vi "GlueSingleModule(SubVI).vi"(0 "XYZ Stage Control":refnum<k24>, 1 "Template Path":path=path "C:/Users/Aerotech/Documents/BNL_ThermomechanicalStave/1_ModulePlacement", 3 "Image Feed":T7, 5 "Module corner coordinates":T3={"X [mm]"=300.0, "Y [mm]"=-149.0, "Z [mm] "=-49.0}, 9 "um/pix resolution":dbl=1.5800403213058958, 11 "error in":errorcluster, 12 "Calibrate distance?":bool, 13 "Tape Type":T2=enum."Left stereo", 14 "Path to save collected images":path=path "C:/Users/Aerotech/cernbox/BNL/Stave Assembly Records/2017-05-12") -> (4 "XYZ .NET Refnum out":refnum<k24>, 15 "error out":errorcluster={"status"=FALSE, "code"=1073676418, "source"="VISA Close in GlueSingleModule(SubVI).vi"})   [LabVIEW 2016]
uses:
  C:/Users/Aerotech/Documents/BNL_ThermomechanicalStave/AerotechLibraries/Bin/Aerotech.A3200.dll
  AerotechLibraries/Bin/Aerotech.A3200.dll
  <vilib>/LabVIEW Interface for Arduino/Type Defs/Arduino Resource.ctl
  <vilib>/LabVIEW Interface for Arduino/Type Defs/Board Type.ctl
  Utils/Enum_TypeDefinitions/Enum_TypeDef_TapeType.ctl
  <vilib>/vision/Image Controls.llb/IMAQ Image.ctl
  <vilib>/LabVIEW Interface for Arduino/Type Defs/Pin Mode.ctl
  <vilib>/Utility/file.llb/Read Delimited Spreadsheet (DBL).vi
  <vilib>/LabVIEW Interface for Arduino/LabVIEW Interface for Arduino.lvlib
panel:
  in  "?":T1(tab)
  in  "Axis speeds (mm/s)":T4={"vX [mm]"=49.0, "vY [mm]"=49.0, "vZ [mm] "=49.0}
  in  "Module length [mm] Y":dbl=90.0
  in  "Module width [mm] X":dbl=90.0
  in  "Home?":bool
  in  "Lowest Z Position":dbl=-47.0
  out "Arduino Resource":T5={"VISA resource"="COM4", "Board Type"=enum."Uno", "Connection Type"=enum."USB / Serial", "Bytes Per Packet (15)"=15}
  in  "Digital I/O Pin":u8=7
  in  "Testing?":bool
  out "Difference camera/syringe in X":dbl
  out "Difference camera/syringe in y":dbl
  in  "Highest Z position":dbl=-49.0
  out "INPUT : Dot":bool[][](array[boolean])
  out "Row":i32
  out "Column":i32
  out "Final Position":T8={"Final X"=300.0000050817871, "Final Y"=-148.9999969595597, "Final Z"=-48.99995500508501}
  out "DY [mm]":dbl[](array[numeric])
  out "DX [mm]":dbl[](array[numeric])
  # "DISPENSE GLUE FOR ONE MODULE  Brandeis University - Brookhaven National Laboratory * ATLAS Phase II Inner Tracker Upgrade"
  # "Overview: This takes a pattern of zeroes/ones (.csv file) as well as the start coordinates of the top left corner of a module and places dots of glue  \nRequirements: NI Arduino dependencies\nInstructions: Select a .csv file (ones indicate regions for glue) as well as a starting coordinate (this is default to the top left corner of the module spacer). You \ncan also input axis speeds (default to maximum) and module lengths and widths (default to 90 mm) which are the widths of the module to which you want to \nplace glue. Lastly, one can choose to Home the stage here and can select the lowest position in Z. The default is that the stage moves down 2-3 mm in Z \nwhile dispensing.  The Arduino inputs are default and simply allow the LabView program to drigger the Arduino (which sends a signal to the dispenser). The \nprogram signals to dispense air- all other parameters such as length of dispensing (default: 350 millisec), pressure (default: 48 psi), and vacuum pressure \n(default: 7.8 psi) are set on the dispenser itself. The defaults are highly recommended here."
  # "Positioning Inputs"
  # "Arduino Inputs"
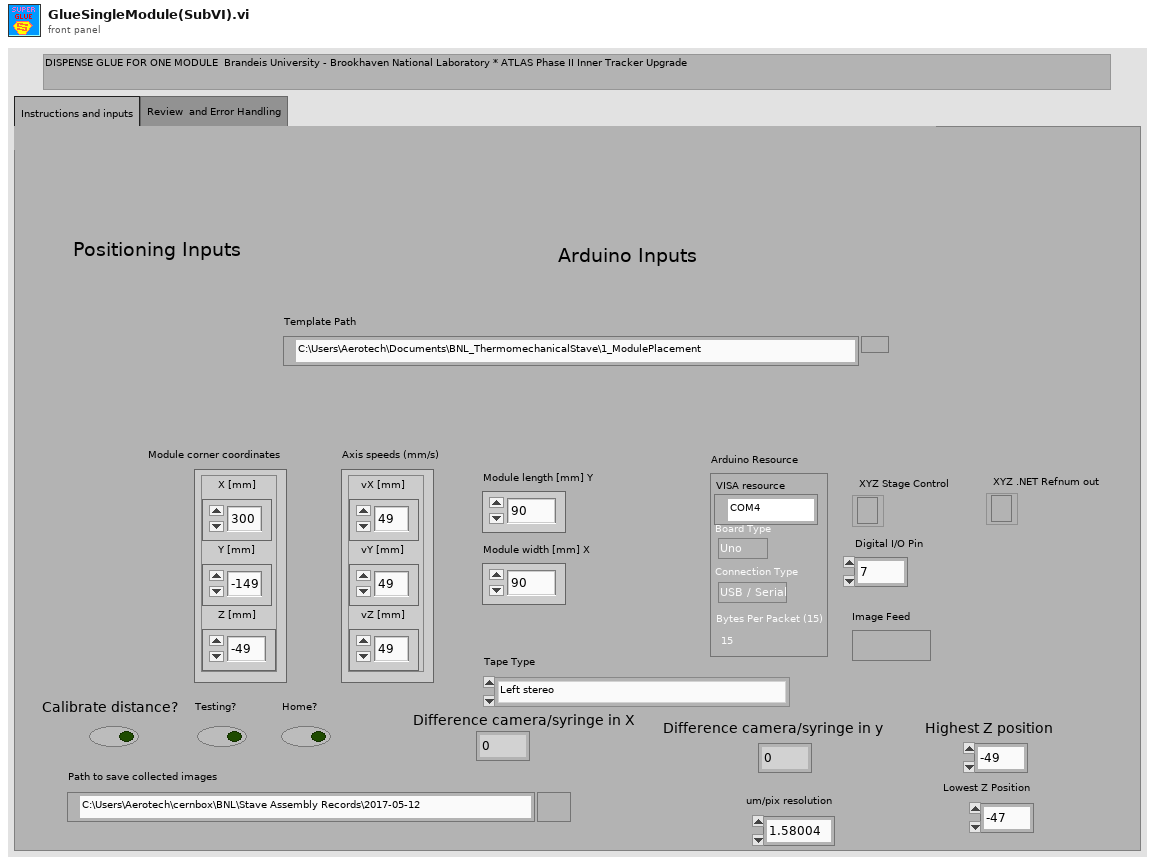
[diagram p1: front panel]
types:
  T1 = enum32{"Instructions and inputs", "Review  and Error Handling"}
  T2 = typedef "Enum_TypeDef_TapeType.ctl" = enum16{"Right stereo", "Left stereo", "Stereo (Sutcliffe NP49-01-100 01-Mar-16)", "Axial (Sutcliffe NP49-01-100 01-Mar-16)"}
  T3 = cluster{"X [mm]":dbl, "Y [mm]":dbl, "Z [mm] ":dbl}
  T4 = cluster{"vX [mm]":dbl, "vY [mm]":dbl, "vZ [mm] ":dbl}
  T5 = typedef "LabVIEW Interface for Arduino.lvlib/Arduino Resource.ctl" = cluster{"VISA resource":refnum<visa-resource-name>, "Board Type":T6, "Connection Type":enum8{"USB / Serial"}, "Bytes Per Packet (15)":u8}
  T6 = typedef "LabVIEW Interface for Arduino.lvlib/Board Type.ctl" = enum16{"Uno", "Dimuelanove w/Atmega 328", "Mega 2560"}
  T7 = typedef "IMAQ Image.ctl" = refnum<image>
  T8 = cluster{"Final X":dbl, "Final Y":dbl, "Final Z":dbl}
  T9 = typedef "LabVIEW Interface for Arduino.lvlib/Pin Mode.ctl" = enum8{"Input", "Output"}
  T10 = cluster{"Final Y":dbl, "Final Y":dbl, "Final Z":dbl}
  T11 = cluster{"Final X":dbl, "Final Y":dbl, "Lowest Z Position":dbl}
  T12 = cluster{"Final X":dbl, "Final Y":dbl, "Z [mm] ":dbl}
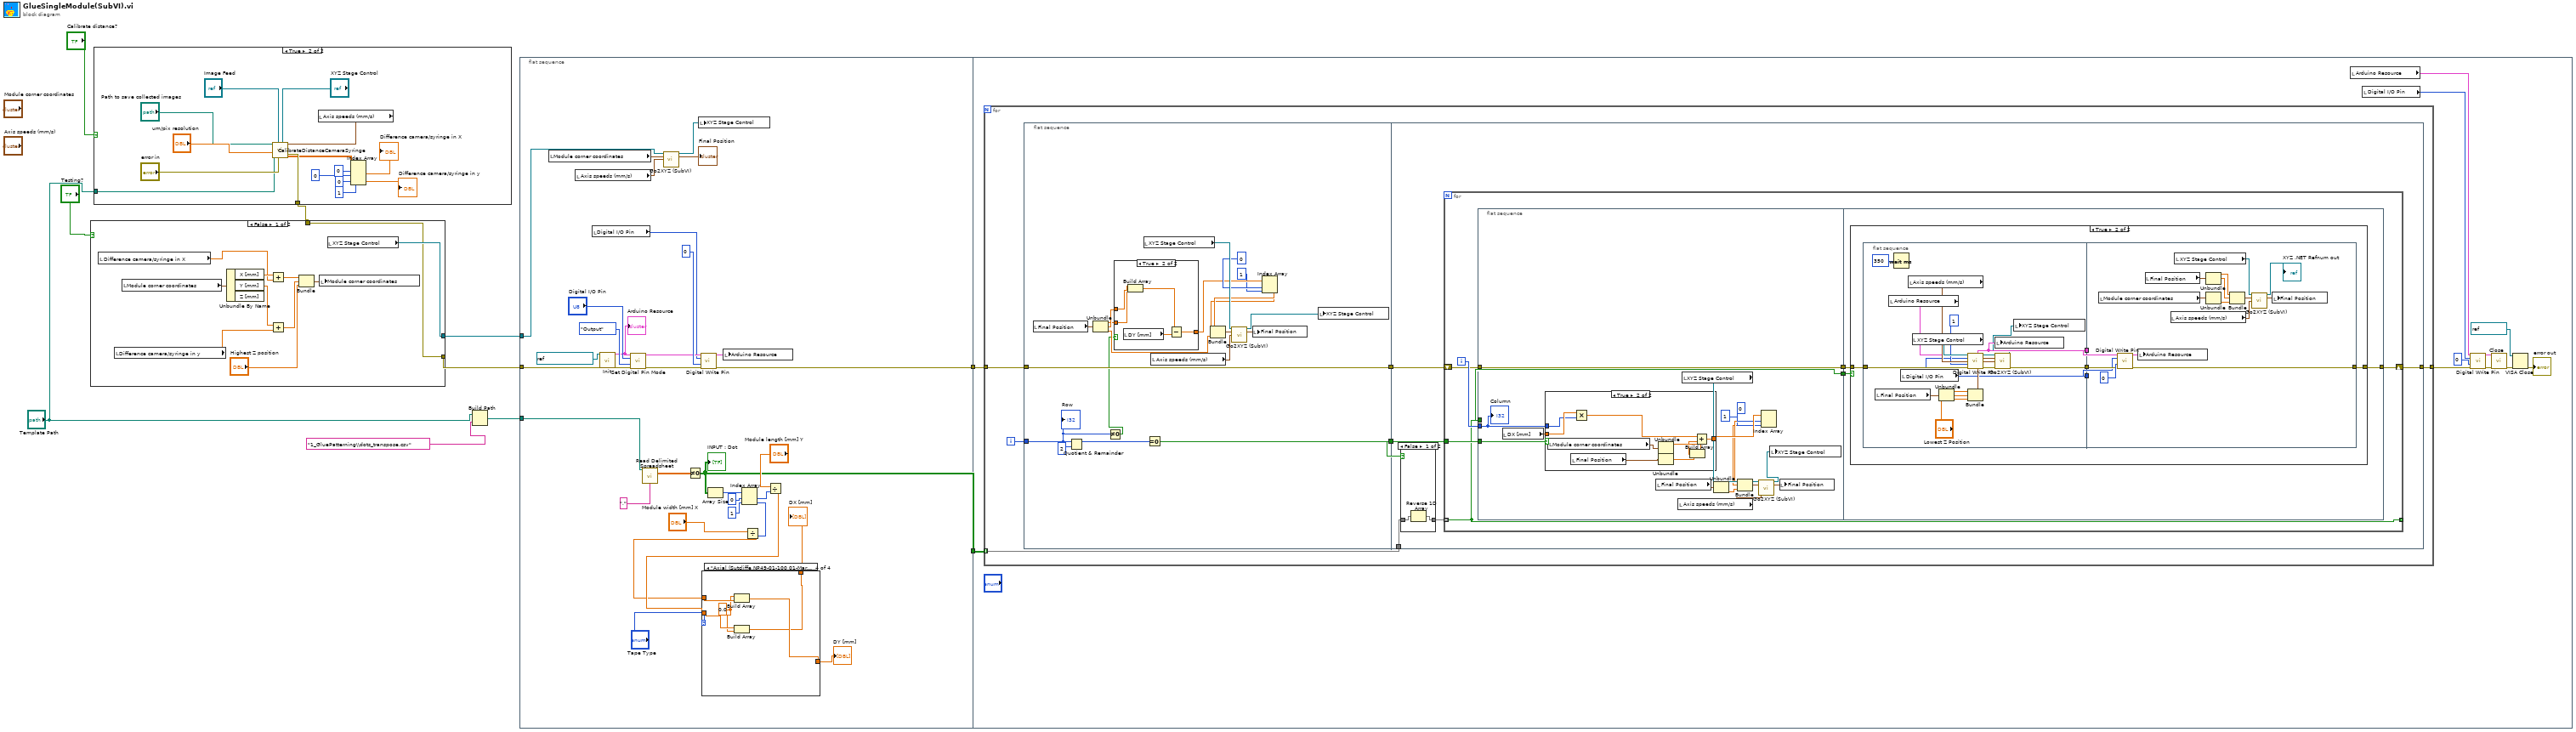
[diagram p0: block diagram]
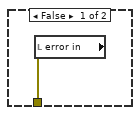
[diagram p2: hidden frame]
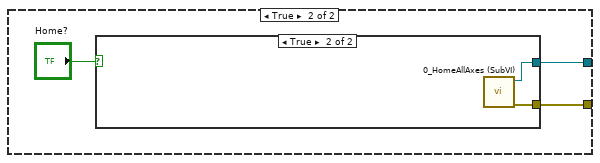
[diagram p3: hidden frame]
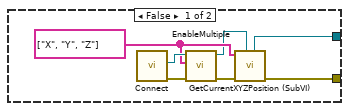
[diagram p4: hidden frame]
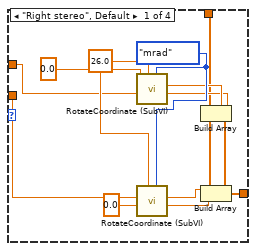
[diagram p5: hidden frame]
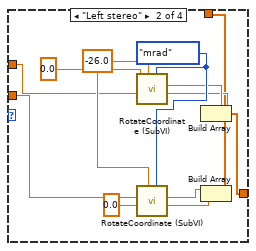
[diagram p6: hidden frame]
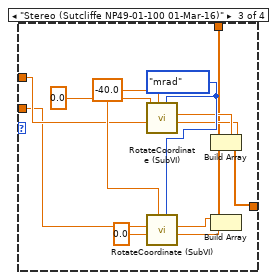
[diagram p7: hidden frame]
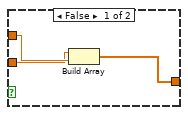
[diagram p8: hidden frame]
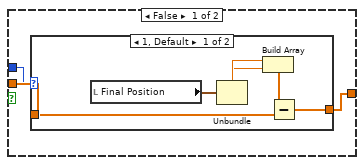
[diagram p10: hidden frame]
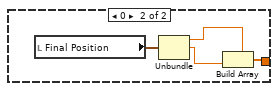
[diagram p11: hidden frame]
diagram:
  n1 = case shown="True" "Calibrate distance?" {
    tunnel: [w11 w22] -> w4
    tunnel: "Template Path" -> [_ w12]
    frame False {
      n2 = local read "error in"() -> (w11:errorcluster)
    }
    frame True {
      n3 = local read "Axis speeds (mm/s)"() -> (w14:T4)
      n4 = call "CalibrateDistanceCameraSyringe.vi"("Axis speeds (mm/s)"=w14, ".NET Refnum in"="XYZ Stage Control", "error in"="error in", "Image Feed"="Image Feed", "Template Path"=w12, "um/pix resolution"="um/pix resolution", "Path to save collected images"="Path to save collected images") -> ("X/Y difference (CAMERA - SYRINGE)"=w21:dbl[][], "error out"=w22:errorcluster)  [unwired: 3 in]
      n5 = Index Array(array=w21, index (row) #1=0 ("index (row)"), index (col) #1=0 ("disabled index (col)"), index (row) #2=0 ("index (row)"), index (col) #2=1 ("disabled index (col)")) -> (element #1=→"Difference camera/syringe in X":dbl, element #2=→"Difference camera/syringe in y":dbl)
    }
  }
  n6 = case shown="False" "Testing?" {
    tunnel: [w28 w39] -> w8
    tunnel: [w27 w38] -> w6
    tunnel: w4 -> [w27 _]
    frame False {
      n7 = local read "Difference camera/syringe in X"() -> (w30:dbl)
      n8 = local read "Difference camera/syringe in y"() -> (w29:dbl)
      n9 = local read "Module corner coordinates"() -> (w37:T3)
      n10 = Unbundle By Name(w37) -> ("X [mm]"=w36:dbl, "Y [mm]"=w35:dbl)  [unwired: 1 out]
      n11 = Add(x=w36, y=w30) -> (x+y=w34:dbl)
      n12 = Add(x=w35, y=w29) -> (x+y=w33:dbl)
      n13 = Bundle(w34, w33, "Highest Z position"="Highest Z position") -> (w32:cluster{dbl, dbl, "Highest Z position":dbl})  [unwired: 1 in]
      n14 = local write "Module corner coordinates"(w32) -> ()
      n15 = local read "XYZ Stage Control"() -> (w28:refnum<k24>)
    }
    frame True {
      n16 = case shown="True" "Home?" {
        tunnel: [w42 w49] -> w39
        tunnel: [w41 w48] -> w38
        frame False {
          w44 = string[] ["X", "Y", "Z"] ("Axes Names")
          n17 = call "Connect.vi"() -> ("error out"=w46:errorcluster, "controller"=w45:refnum<k24>)  [unwired: 10 in]
          n18 = call "EnableMultiple.vi"("error in (no error)"=w46, "axis names"=w44, "controller in"=w45) -> ("error out"=w47:errorcluster, "controller out"=w43:refnum<k24>)  [unwired: 7 in]
          n19 = call "GetCurrentXYZPosition (SubVI).vi"(".NET Refnum in - Device"=w43, "error in (no error)"=w47, "Axes Names"=w44) -> ("error out"=w41:errorcluster, ".NET Refnum out  - Device"=w42:refnum<k24>)  [unwired: 3 in, 4 out]
        }
        frame True {
          n20 = call "0_HomeAllAxes (SubVI).vi"() -> ("error out"=w48:errorcluster, "controller out"=w49:refnum<k24>)  [unwired: 8 in, 2 out]
        }
      }
    }
  }
  n21 = Build Path(base path="Template Path", name or relative path="1_GluePatterning\\dots_transpose.csv") -> (appended path=w1:path)
  n22 = flat-sequence {
    tunnel: [w82] -> w10
    tunnel: [w60] -> w9
    tunnel: w8 -> [w57]
    tunnel: w6 -> [w56]
    tunnel: w1 -> [w50]
    tunnel: w10 -> [w134]
    tunnel: w9 -> [w133]
    frame #0 {
      n23 = local read "Module corner coordinates"() -> (w70:T3)
      n24 = local read "Axis speeds (mm/s)"() -> (w72:T4)
      n25 = local read "Digital I/O Pin"() -> (w62:u8)
      n26 = call <vilib>:"Init.vi"("VISA resource"=refnum<visa-resource-name> "COM4", "error in"=w56) -> ("Arduino Resource"=w61:T5, "error out"=w63:errorcluster)  [unwired: 16 in]
      "Arduino Resource" <- w61
      n27 = call <vilib>:"Set Digital Pin Mode.vi"("Arduino Resource"=w61, "Digital I/O Pin"="Digital I/O Pin", "Pin Mode (Input)"=Pin_Mode."Output", "error in"=w63) -> ("Arduino Resource"=w66:T5, "error out"=w67:errorcluster)  [unwired: 10 in]
      n28 = call-poly <vilib>:"Read Delimited Spreadsheet.vi"("file path (dialog if empty)"=w50, "delimiter (\\t)"="," ("delimiter (\\t)")) -> ("all rows"=w80:dbl[][])  [unwired: 8 in, 5 out]
      n29 = call "Go2XYZ (SubVI).vi"(".NET Refnum in"=w57, "Go to Coordinates"=w70, "Axis Speeds"=w72) -> (".NET Refnum out"=w71:refnum<k24>, "Final Position"=→"Final Position":T8)  [unwired: 8 in, 3 out]
      n30 = Not Equal To 0?(x=w80) -> (x != 0?=w60:bool[][])
      "INPUT : Dot" <- w60
      n31 = local write "XYZ Stage Control"(w71) -> ()
      n32 = call <vilib>:"Digital Write Pin.vi"("Arduino Resource"=w66, "Digital I/O Pin (0)"=w62, "Value (0)"=u8 0, "error in"=w67) -> ("Arduino Resource"=w58:T5, "error out"=w82:errorcluster)  [unwired: 10 in]
      n33 = Array Size(array=w60) -> (size(s)=w79:i32[])
      n34 = local write "Arduino Resource"(w58) -> ()
      n35 = Index Array(array=w79, index #1=0 ("index"), index #2=1 ("index")) -> (element #1=w75:i32, element #2=w74:i32)
      n36 = Divide(x="Module width [mm] X", y=w74) -> (x/y=w51:dbl)
      n37 = Divide(x="Module length [mm] Y", y=w75) -> (x/y=w52:dbl)
      n38 = case shown="\"Axial (Sutcliffe NP49-01-100 01-Mar-16)\"" "Tape Type" {
        tunnel: w52 -> [w90 w97 w109 w123]
        tunnel: w51 -> [w92 w98 w110 w122]
        tunnel: [w83 w96 w107 w119] -> w54
        tunnel: [w84 w95 w108 w120] -> w53
        frame "Right stereo", Default {
          w93 = 26.0 ("Angle")
          w94 = enum16{"mrad", "Radians", "Degrees"}."mrad" ("Units")
          n39 = call "RotateCoordinate (SubVI).vi"("Units"=w94, "Angle"=w93, "y"=w92, "x"=0.0) -> ("y'"=w87:dbl, "x'"=w88:dbl)  [unwired: 5 in, 1 out]
          n40 = call "RotateCoordinate (SubVI).vi"("Units"=w94, "Angle"=w93, "y"=0.0, "x"=w90) -> ("y'"=w85:dbl, "x'"=w86:dbl)  [unwired: 5 in, 1 out]
          n41 = Build Array(w88, w87) -> (w84:dbl[])
          n42 = Build Array(w86, w85) -> (w83:dbl[])
        }
        frame "Left stereo" {
          w105 = -26.0 ("Angle")
          w106 = enum16{"mrad", "Radians", "Degrees"}."mrad" ("Units")
          n43 = call "RotateCoordinate (SubVI).vi"("Units"=w106, "Angle"=w105, "y"=w98, "x"=0.0) -> ("y'"=w101:dbl, "x'"=w102:dbl)  [unwired: 5 in, 1 out]
          n44 = call "RotateCoordinate (SubVI).vi"("Units"=w106, "Angle"=w105, "y"=0.0, "x"=w97) -> ("y'"=w99:dbl, "x'"=w100:dbl)  [unwired: 5 in, 1 out]
          n45 = Build Array(w102, w101) -> (w95:dbl[])
          n46 = Build Array(w100, w99) -> (w96:dbl[])
        }
        frame "Stereo (Sutcliffe NP49-01-100 01-Mar-16)" {
          w117 = -40.0 ("Angle")
          w118 = enum16{"mrad", "Radians", "Degrees"}."mrad" ("Units")
          n47 = call "RotateCoordinate (SubVI).vi"("Units"=w118, "Angle"=w117, "y"=w110, "x"=0.0) -> ("y'"=w113:dbl, "x'"=w114:dbl)  [unwired: 5 in, 1 out]
          n48 = call "RotateCoordinate (SubVI).vi"("Units"=w118, "Angle"=w117, "y"=0.0, "x"=w109) -> ("y'"=w111:dbl, "x'"=w112:dbl)  [unwired: 5 in, 1 out]
          n49 = Build Array(w114, w113) -> (w108:dbl[])
          n50 = Build Array(w112, w111) -> (w107:dbl[])
        }
        frame "Axial (Sutcliffe NP49-01-100 01-Mar-16)" {
          w121 = 0.0 ("element")
          n51 = Build Array(w121, w122) -> (w120:dbl[])
          n52 = Build Array(w123, w121) -> (w119:dbl[])
        }
      }
      "DX [mm]" <- w54
      "DY [mm]" <- w53
    }
    frame #1 {
      n53 = for {
        tunnel: w133 -> [w135] mode=indexing
        tunnel: [w139] -> w126
        tunnel: w134 -> [w137]
        i -> [w140]
        n54 = flat-sequence {
          tunnel: w140 -> [w149]
          tunnel: [w160] -> w138
          tunnel: w137 -> [w160]
          tunnel: [w151] -> w136
          tunnel: w135 -> [w171]
          tunnel: [w173] -> w139
          tunnel: w138 -> [w172]
          tunnel: w136 -> [w169]
          frame #0 {
            n55 = local read "Final Position"() -> (w156:T8)
            n56 = Quotient & Remainder(x=w149, y=2) -> (x-y*floor(x/y)=w152:i32)  [unwired: 1 out]
            n57 = Unbundle(w156) -> ("Final X"=w143:dbl, "Final Y"=w158:dbl, "Final Z"=w157:dbl)
            n58 = Not Equal To 0?(x=w149) -> (x != 0?=w148:bool)
            n59 = case shown="True" w148 {
              tunnel: [w163 w168] -> w146
              tunnel: w158 -> [w162 w166]
              tunnel: w143 -> [w161 w164]
              frame False {
                n60 = Build Array(w161, w162) -> (w163:dbl[])
              }
              frame True {
                n61 = local read "DY [mm]"() -> (w167:dbl[])
                n62 = Build Array(w164, w166) -> (w165:dbl[])
                n63 = Subtract(x=w165, y=w167) -> (x-y=w168:dbl[])
              }
            }
            n64 = local read "XYZ Stage Control"() -> (w154:refnum<k24>)
            n65 = Equal To 0?(x=w152) -> (x = 0?=w151:bool)
            n66 = local read "Axis speeds (mm/s)"() -> (w159:T4)
            n67 = Index Array(array=w146, index #1=0 ("index"), index #2=1 ("index")) -> (element #1=w145:dbl, element #2=w144:dbl)
            n68 = Bundle("Final Y"=w145, "Final Y"=w144, "Final Z"=w157) -> (w155:T10)  [unwired: 1 in]
            n69 = call "Go2XYZ (SubVI).vi"(".NET Refnum in"=w154, "Go to Coordinates"=w155, "Axis Speeds"=w159) -> (".NET Refnum out"=w141:refnum<k24>, "Final Position"=w153:T8)  [unwired: 8 in, 3 out]
            n70 = local write "Final Position"(w153) -> ()
            n71 = local write "XYZ Stage Control"(w141) -> ()
            "Row" <- w149
          }
          frame #1 {
            n72 = case shown="False" w169 {
              tunnel: w171 -> [w175 w176]
              tunnel: [w174 w176] -> w170
              frame False {
                n73 = Reverse 1D Array(array=w175) -> (reversed array=w174:bool[])
              }
              frame True {
              }
            }
            n74 = for {
              shift-right: [w179] -> w173
              shift-left: w172 -> [w182]
              tunnel: [w177] -> _ mode=indexing
              tunnel: w169 -> [w178]
              tunnel: w170 -> [w177] mode=indexing
              i -> [w183]
              n75 = flat-sequence {
                tunnel: [w196] -> w181
                tunnel: [w190] -> w180
                tunnel: w183 -> [w197]
                tunnel: w182 -> [w196]
                tunnel: w177 -> [w190]
                tunnel: w178 -> [w191]
                tunnel: w181 -> [w225]
                tunnel: w180 -> [w223]
                tunnel: [w224] -> w179
                frame #0 {
                  n76 = local read "DX [mm]"() -> (w198:dbl[])
                  n77 = case shown="True" w191 {
                    tunnel: w198 -> [w202 w222]
                    tunnel: w197 -> [w201 w219]
                    tunnel: [w203 w220] -> w189
                    frame False {
                      n78 = case shown="1, Default" w201 {
                        tunnel: [w209 w210] -> w203
                        tunnel: w202 -> [w208 _]
                        frame 1, Default {
                          n79 = local read "Final Position"() -> (w207:T8)
                          n80 = Unbundle(w207) -> ("Final X"=w206:dbl, "Final Y"=w205:dbl)  [unwired: 1 out]
                          n81 = Build Array(w206, w205) -> (w204:dbl[])
                          n82 = Subtract(x=w204, y=w208) -> (x-y=w209:dbl[])
                        }
                        frame 0 {
                          n83 = local read "Final Position"() -> (w213:T8)
                          n84 = Unbundle(w213) -> ("Final X"=w212:dbl, "Final Y"=w211:dbl)  [unwired: 1 out]
                          n85 = Build Array(w212, w211) -> (w210:dbl[])
                        }
                      }
                    }
                    frame True {
                      n86 = local read "Module corner coordinates"() -> (w216:T3)
                      n87 = local read "Final Position"() -> (w215:T8)
                      n88 = Multiply(x=w222, y=w219) -> (x*y=w221:dbl[])
                      n89 = Unbundle(w216) -> ("X [mm]"=w218:dbl)  [unwired: 2 out]
                      n90 = Unbundle(w215) -> ("Final Y"=w214:dbl)  [unwired: 2 out]
                      n91 = Build Array(w218, w214) -> (w217:dbl[])
                      n92 = Add(x=w221, y=w217) -> (x+y=w220:dbl[])
                    }
                  }
                  n93 = local read "Final Position"() -> (w195:T8)
                  n94 = local read "Axis speeds (mm/s)"() -> (w200:T4)
                  n95 = local read "XYZ Stage Control"() -> (w199:refnum<k24>)
                  n96 = Unbundle(w195) -> ("Final Z"=w192:dbl)  [unwired: 2 out]
                  n97 = Index Array(array=w189, index #1=0 ("index"), index #2=1 ("index")) -> (element #1=w186:dbl, element #2=w185:dbl)
                  n98 = Bundle("Final Y"=w186, "Final Y"=w185, "Final Z"=w192) -> (w193:T10)  [unwired: 1 in]
                  n99 = call "Go2XYZ (SubVI).vi"(".NET Refnum in"=w199, "Go to Coordinates"=w193, "Axis Speeds"=w200) -> (".NET Refnum out"=w184:refnum<k24>, "Final Position"=w194:T8)  [unwired: 8 in, 3 out]
                  n100 = local write "XYZ Stage Control"(w184) -> ()
                  n101 = local write "Final Position"(w194) -> ()
                  "Column" <- w197
                }
                frame #1 {
                  n102 = case shown="True" w223 {
                    tunnel: [w226 w231] -> w224
                    tunnel: w225 -> [w226 w229]
                    frame False {
                    }
                    frame True {
                      n103 = flat-sequence {
                        tunnel: [w240] -> w230
                        tunnel: w229 -> [w237]
                        tunnel: [w234] -> w228
                        tunnel: [w233] -> w227
                        tunnel: [w252] -> w231
                        tunnel: w230 -> [w253]
                        tunnel: w228 -> [w251]
                        tunnel: w227 -> [w250]
                        frame #0 {
                          n104 = local read "Final Position"() -> (w243:T8)
                          n105 = local read "Arduino Resource"() -> (w239:T5)
                          n106 = Wait (ms)(milliseconds to wait=u32 350) -> ()  [unwired: 1 out]
                          n107 = local read "Digital I/O Pin"() -> (w234:u8)
                          n108 = local read "Axis speeds (mm/s)"() -> (w246:T4)
                          n109 = local read "XYZ Stage Control"() -> (w245:refnum<k24>)
                          n110 = Unbundle(w243) -> ("Final X"=w242:dbl, "Final Y"=w241:dbl)  [unwired: 1 out]
                          n111 = call <vilib>:"Digital Write Pin.vi"("Arduino Resource"=w239, "Digital I/O Pin (0)"=w234, "Value (0)"=u8 1, "error in"=w237) -> ("Arduino Resource"=w233:T5, "error out"=w236:errorcluster)  [unwired: 10 in]
                          n112 = Bundle("Final X"=w242, "Final Y"=w241, "Lowest Z Position"="Lowest Z Position") -> (w244:T11)  [unwired: 1 in]
                          n113 = local write "Arduino Resource"(w233) -> ()
                          n114 = call "Go2XYZ (SubVI).vi"(".NET Refnum in"=w245, "Go to Coordinates"=w244, "Axis Speeds"=w246, "error in (no error)"=w236) -> (".NET Refnum out"=w232:refnum<k24>, "error out"=w240:errorcluster)  [unwired: 7 in, 3 out]
                          n115 = local write "XYZ Stage Control"(w232) -> ()
                        }
                        frame #1 {
                          n116 = local read "Module corner coordinates"() -> (w262:T3)
                          n117 = call <vilib>:"Digital Write Pin.vi"("Arduino Resource"=w250, "Digital I/O Pin (0)"=w251, "Value (0)"=u8 0, "error in"=w253) -> ("Arduino Resource"=w249:T5, "error out"=w252:errorcluster)  [unwired: 10 in]
                          n118 = local write "Arduino Resource"(w249) -> ()
                          n119 = local read "Final Position"() -> (w263:T8)
                          n120 = local read "Axis speeds (mm/s)"() -> (w257:T4)
                          n121 = local read "XYZ Stage Control"() -> (w256:refnum<k24>)
                          n122 = Unbundle(w263) -> ("Final X"=w261:dbl, "Final Y"=w260:dbl)  [unwired: 1 out]
                          n123 = Unbundle(w262) -> ("Z [mm]"=w259:dbl)  [unwired: 2 out]
                          n124 = Bundle("Final X"=w261, "Final Y"=w260, "Z [mm]"=w259) -> (w258:T12)  [unwired: 1 in]
                          n125 = call "Go2XYZ (SubVI).vi"(".NET Refnum in"=w256, "Go to Coordinates"=w258, "Axis Speeds"=w257) -> (".NET Refnum out"=→"XYZ .NET Refnum out":refnum<k24>, "Final Position"=w255:T8)  [unwired: 8 in, 3 out]
                          n126 = local write "Final Position"(w255) -> ()
                        }
                      }
                    }
                  }
                }
              }
            }
          }
        }
      }
      n127 = local read "Arduino Resource"() -> (w130:T5)
      n128 = local read "Digital I/O Pin"() -> (w131:u8)
      n129 = call <vilib>:"Digital Write Pin.vi"("Arduino Resource"=w130, "Digital I/O Pin (0)"=w131, "Value (0)"=u8 0, "error in"=w126) -> ("Arduino Resource"=w128:T5, "error out"=w127:errorcluster)  [unwired: 10 in]
      n130 = call <vilib>:"Close.vi"("Arduino Resource"=w128, "error in"=w127) -> ("error out"=w125:errorcluster)  [unwired: 13 in]
      n131 = VISA Close(VISA resource name=refnum<visa-resource-name> "COM3", error in (no error)=w125) -> (error out=→"error out":errorcluster)
    }
  }
